vi "DiffDriveOdom_ExecRelativeTraj.vi"(11 "Init":bool) -> (1 "AtReference":bool, 2 "Right Speed Target":dbl, 3 "Left Speed Target":dbl)   [LabVIEW 2019]
uses:
  <vilib>/Rock Robotics/WPI/ThirdParty/JAS_Junk/TrajLib/VI/numCmd_ObtainQueue_Array.vi
  <vilib>/Rock Robotics/WPI/ThirdParty/JAS_Junk/TrajLib/Trajectory_Library.lvlib
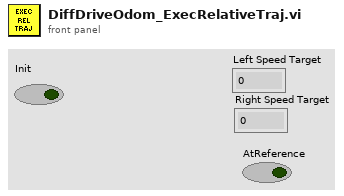
[diagram p1: front panel]
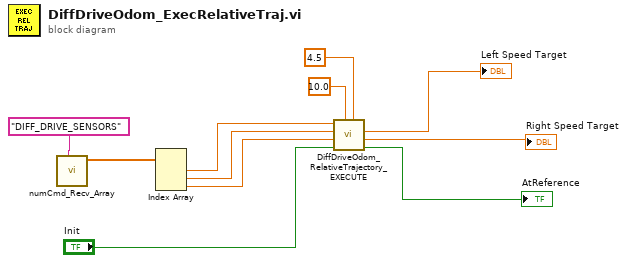
[diagram p0: block diagram]
diagram:
  n1 = call <vilib>:"numCmd_Recv_Array.vi"("Command Name"="DIFF_DRIVE_SENSORS") -> ("Values"=w8:dbl[])  [unwired: 8 in, 2 out]
  n2 = Index Array(array=w8) -> (element #1=w7:dbl, element #2=w6:dbl, element #3=w5:dbl)  [unwired: 3 in]
  n3 = call "DiffDriveOdom_RelativeTrajectory_EXECUTE.vi"("Track Width FT"=4.5, "Max Speed\nFT/SEC"=10.0 ("Max Speed\nFT/SEC"), "Init"="Init", "Gyro Continous\n (inc counterclockwise)\nDEG"=w5, "Right Distance FT"=w6, "Left Distance FT"=w7) -> ("AtReference"=→"AtReference":bool, "Right Speed Target"=→"Right Speed Target":dbl, "Left Speed Target"=→"Left Speed Target":dbl)  [unwired: 3 in]
